vi "Channels.Inline.Read.Channel Block Descriptor (Single).vi"(8 "error in (no error)":errorcluster, 10 "Values Array in":dbl[](array[numeric]), 11 "Channel Block Descriptor":T1) -> (0 "error out":errorcluster, 2 "Values Array out":dbl[](array[numeric]), 3 "Channel Block Descriptor dup":T1)   [LabVIEW 2016, in "VeriStand Data.lvlib"]
doc: "Reads the block of channel data specified by <B>Channel Block Descriptor</B> into the provided <B>Values Array</B>."
uses:
  VeriStand Data.lvlib
  Typedefs/Typedefs.Block Descriptor.Channel Block.ctl
  Typedefs/Typedefs.Block Descriptor.ctl
  Memory Management/Memory Management.Handle Return.vi
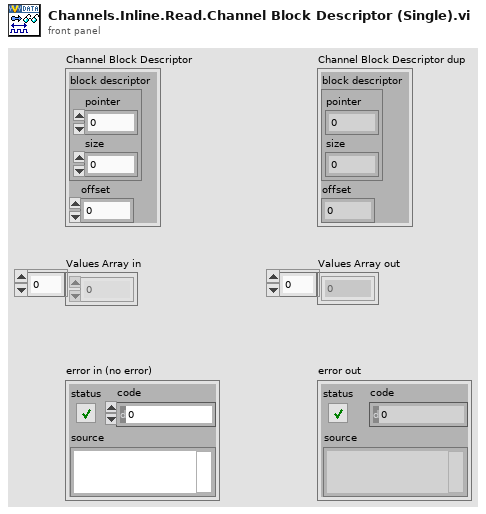
[diagram p1: front panel]
types:
  T1 = typedef "VeriStand Data.lvlib/Typedefs.Block Descriptor.Channel Block.ctl" = cluster{"block descriptor":T2, "offset":u64}
  T2 = typedef "VeriStand Data.lvlib/Typedefs.Block Descriptor.ctl" = cluster{"pointer":u64, "size":i64}
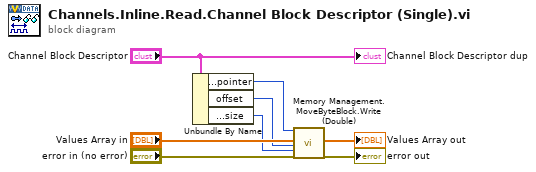
[diagram p0: block diagram]
diagram:
  n1 = Unbundle By Name("Channel Block Descriptor") -> ("block descriptor.pointer"=w2:u64, "offset"=w3:u64, "block descriptor.size"=w4:i64)
  n2 = call "Memory Management.MoveByteBlock.Write (Double).vi"("src ptr in"=w2, "dst in"="Values Array in", "dst offset (0)"=w3, "size"=w4, "error in (no error)"="error in (no error)") -> ("dst out"=→"Values Array out":dbl[], "error out"=→"error out":errorcluster)  [unwired: 9 in, 4 out]
  "Channel Block Descriptor dup" <- "Channel Block Descriptor"
